vi "Msg EnQ.vi"(9 "Msg":refnum<class "Msg.lvclass">, 10 "Msg Q":refnum<class "Msg Q.lvclass">, 11 "Priority Msg EnQ in":refnum<class "Priority Msg EnQ.lvclass">) -> (0 "error out":errorcluster)   [LabVIEW 2021, in "AAM.lvlib" / "Priority Msg EnQ.lvclass"]
uses:
  Priority Msg EnQ.lvclass
  Msg/Msg.lvclass
  Msg Q/Msg Q.lvclass
  Msg Q/Msg Q.lvclass/Msg Q.ctl
  Msg Q/Read Msg Q.vi
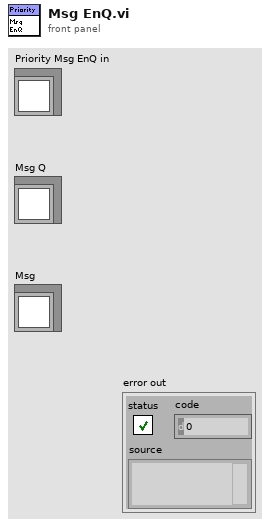
[diagram p1: front panel]
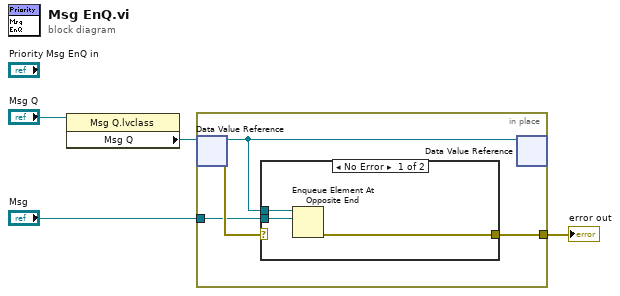
[diagram p0: block diagram]
diagram:
  n1 = property class="Msg Q.lvclass"(reference="Msg Q") -> ("Msg Q"=w4:refnum<data-value>)  [unwired: 1 in, 2 out]
  n2 = in-place {
    in-place-border: [w7] -> w1
    in-place-border: "Msg" -> [w6]
    n3 = in-place-dvr #1(w4) -> (w5:refnum<queue>, w8:errorcluster)
    n4 = case shown="No Error" w8 {
      selector: w8 -> [_ w12]
      tunnel: [w11 w12] -> w7
      tunnel: w6 -> [w10 _]
      tunnel: w5 -> [w9 _]
      frame No Error {
        n5 = Enqueue Element At Opposite End(queue=w9, element=w10) -> (error out=w11:errorcluster)  [unwired: 2 in, 2 out]
      }
      frame Error {
      }
    }
    n6 = in-place-dvr #1(w5) -> ()  [unwired: 2 out]
  }
  "error out" <- w1
